vi "Express VI.vi"() -> ()   [LabVIEW 2023]
uses:
  <vilib>/express/express arith-compare/Formula/XNode/ExpressFormulaBlockNode.xnode
panel:
  out "结果":dbl
  in  "stop":bool
  in  "X1":dbl
  in  "X2":dbl
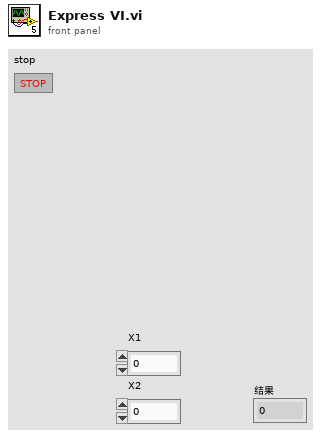
[diagram p1: front panel]
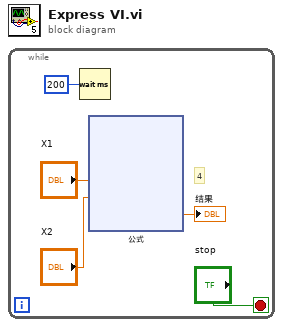
[diagram p0: block diagram]
diagram:
  n1 = while {
    stop <- "stop" stop-if-true
    # "4"
    n2 = Wait (ms)(milliseconds to wait=u32 200 ("millisecond timer value")) -> ()  [unwired: 1 out]
    n3 = xnode "公式"("X1"="X1", "X2"="X2") -> ("Result"=→"结果":dbl)  [unwired: 1 in, 1 out]
  }
